vi "DSB Modulation Demo (Baseband-Sine) - PLL.vi"() -> ()   [LabVIEW 2013]
uses:
  <vilib>/addons/Modulation/Analog/MT Passband PLL.vi
  <vilib>/express/express analysis/Spectral/Block/exnSpectralBlock spectral measurements RMS poly.vi
  <vilib>/express/express analysis/Spectral/Block/exnSpectralBlock spectral measurements RMS DDT.vi
  <vilib>/express/express analysis/Spectral/XNode/ExpressSpectralMeasurementsBlockNode.xnode
  <vilib>/addons/Modulation/niAMT.lvlib
panel:
  out "Esitimated Freq":dbl
  in  "Modulation Freq.":dbl=2000.0 caption="Frequency"
  in  "?":enum32{"DSB FFT", "DSB Squared"}(tab)
  out "DSB FFT":dynamicdata(graph)
  out "DSB Squared":dynamicdata(graph)
  in  "WAV Sample Rate":dbl=44100.0 caption="dt"
  in  "LPF Cut-Off":dbl=10000.0 caption="Lower Cut-Off"
  in  "SNR (dB)":dbl(slide)=30.0 caption="Standard deviation" scale=-20.0..30.0
  out "Comparision":dynamicdata(graph)
  out "Baseband":dynamicdata(graph)
  out "DSB Wave":dynamicdata(graph)
  in  "Carrier Amp.":dbl=1.0 caption="Amplitude"
  in  "stop":bool
  in  "Frequency Offset":dbl(slide) scale=0.0..1000.0
  in  "Carrier Freq.":dbl=100000.0 caption="Frequency"
  # "DSB Modulation"
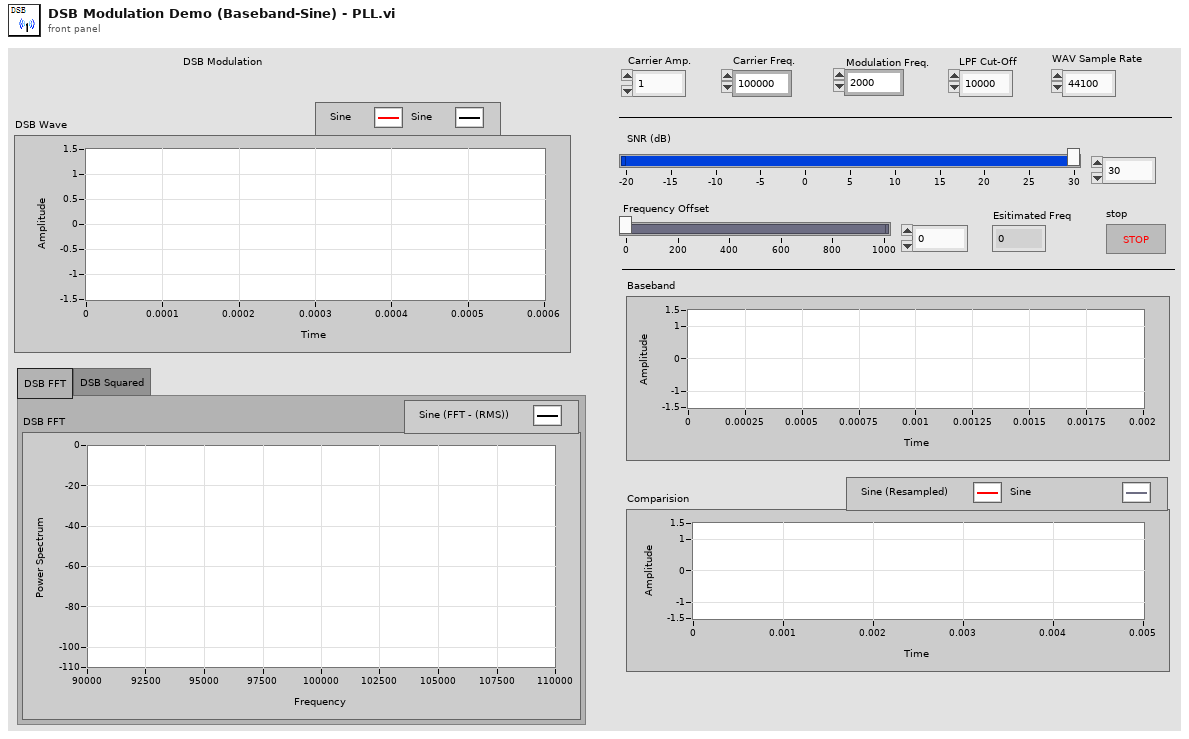
[diagram p1: front panel]
types:
  T1 = cluster{"averaging mode":u16, "weighting mode":u16, "number of averages":u32}
  T2 = cluster{"dB On (F)":bool, "unwrap phase (F)":bool, "convert to degree (F)":bool}
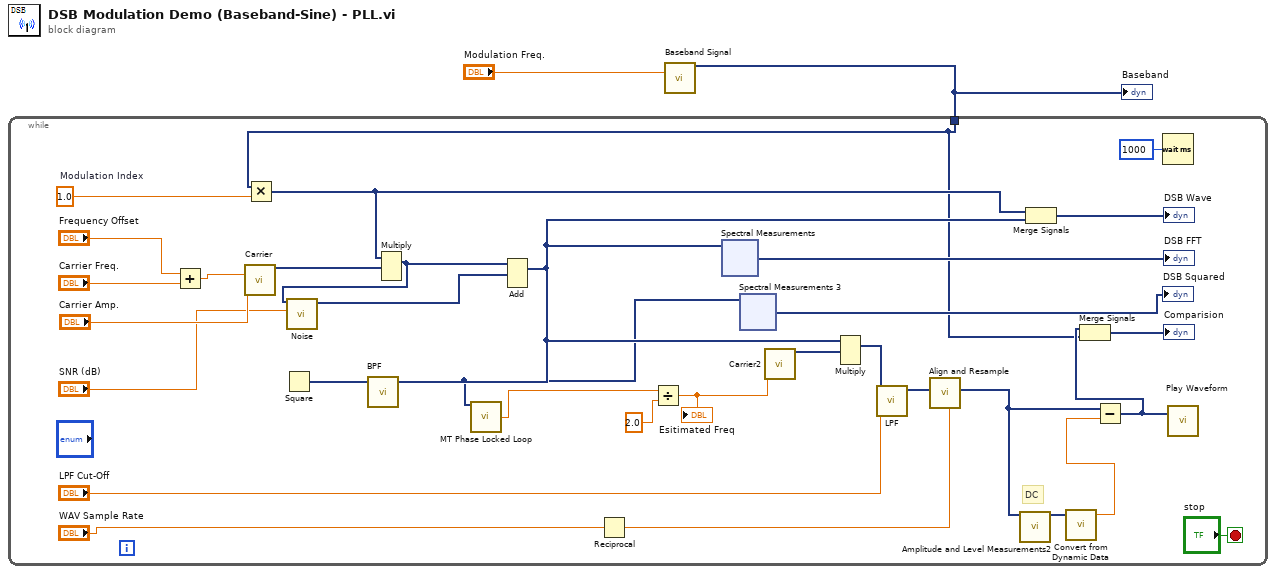
[diagram p0: block diagram]
diagram:
  n1 = call "Baseband Signal"("Frequency"="Modulation Freq.") -> ("Sine"=w1:dynamicdata)  [unwired: 13 in, 1 out]
  "Baseband" <- w1
  n2 = while {
    tunnel: w1 -> [w3]
    stop <- "stop" stop-if-true
    w29 = 1.0  # Modulation Index
    # "DC"
    n3 = Add(x="Frequency Offset", y="Carrier Freq.") -> (x+y=w28:dbl)
    n4 = call "Carrier"("Frequency"=w28, "Amplitude"="Carrier Amp.") -> ("Sine"=w26:dynamicdata)  [unwired: 12 in, 1 out]
    n5 = Multiply(x=w3, y=w29) -> (x*y=w25:dynamicdata)
    n6 = Multiply(1:w26, 2:w25) -> (0:w12:dynamicdata)  [unwired: 1 in, 1 out]
    n7 = call "Noise.vi"("AWGN (dB)"="SNR (dB)", "Dynamic Data"=w12) -> ("DC with Gaussian Noise"=w24:dynamicdata)  [unwired: 9 in]
    n8 = Add(1:w24, 2:w12) -> (0:w11:dynamicdata)  [unwired: 1 in, 1 out]
    n9 = Square(x=w11) -> (x^2=w10:dynamicdata)
    n10 = call "BPF"("Signal"=w10) -> ("Filtered Signal"=w5:dynamicdata)  [unwired: 9 in, 1 out]
    n11 = call-poly <vilib>:"MT Phase Locked Loop.vi"("passband waveform"=w5) -> ("estimated carrier frequency (Hz)"=w4:dbl)  [unwired: 10 in, 4 out]
    n12 = Reciprocal(x="WAV Sample Rate") -> (1/x=w13:dbl)
    n13 = Divide(x=w4, y=2.0) -> (x/y=w6:dbl)
    "Esitimated Freq" <- w6
    n14 = xnode "Spectral Measurements"("Signals"=w11) -> ("FFT - (RMS)"=→"DSB FFT":dynamicdata)  [unwired: 2 in, 3 out]
    n15 = xnode "Spectral Measurements 3"("Signals"=w5) -> ("FFT - (RMS)"=→"DSB Squared":dynamicdata)  [unwired: 2 in, 3 out]
    n16 = call "Carrier2"("Frequency"=w6) -> ("Sine"=w21:dynamicdata)  [unwired: 13 in, 1 out]
    n17 = Multiply(1:w21, 2:w11) -> (0:w20:dynamicdata)  [unwired: 1 in, 1 out]
    n18 = call "LPF"("Lower Cut-Off"="LPF Cut-Off", "Signal"=w20) -> ("Filtered Signal"=w19:dynamicdata)  [unwired: 8 in, 1 out]
    n19 = call "Align and Resample"("dt"=w13, "Signals"=w19) -> ("Resampled Signals"=w32:dynamicdata)  [unwired: 7 in, 2 out]
    n20 = call "Amplitude and Level Measurements2"("Signals"=w32) -> ("Mean (DC)"=w34:dynamicdata)  [unwired: 13 in, 1 out]
    n21 = Merge Signals(w25, w11) -> (→"DSB Wave":dynamicdata)
    n22 = call "Convert from Dynamic Data"("Dynamic Data Type"=w34) -> ("Scalar"=w31:dbl)  [unwired: 3 in]
    n23 = Subtract(x=w32, y=w31) -> (x-y=w17:dynamicdata)
    n24 = Merge Signals(w17, w3) -> (→"Comparision":dynamicdata)
    n25 = Wait (ms)(milliseconds to wait=u32 1000) -> ()  [unwired: 1 out]
    n26 = call "Play Waveform"("Data"=w17) -> ()  [unwired: 18 in, 1 out]
  }
